vi "sub_generate-ray-casting-grid-map.vi"() -> ()   [LabVIEW 2019]
uses:
  Ctrl/cmd_common.ctl
panel:
  out "oy":dbl[](array[numeric])
  out "ox":dbl[](array[numeric])
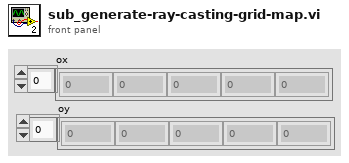
[diagram p1: front panel]
types:
  T1 = typedef "cmd_common.ctl" = enum16{"read", "write"}
  T2 = typedef "NI_Matrix.lvlib/RealMatrix.ctl" = dbl[][]
  T3 = cluster{"resolution":dbl, "EXTEND_AREA":dbl, "MAX_RANGE":dbl, "NP":u32, "NTh":u32, "Q":T2, "R":T2, "Q_sim":T2, "R_sim":T2, "rf_id":cluster{"x":dbl, "y":dbl}[]}
  T4 = cluster{"ox":T2, "oy":T2, "occupancy map":T2, "x_true":T2, "u":T2, "z":T2, "PEst":T2, "min x":dbl, "min y":dbl, "max x":dbl, "max y":dbl, "yw":i32, "xw":i32}
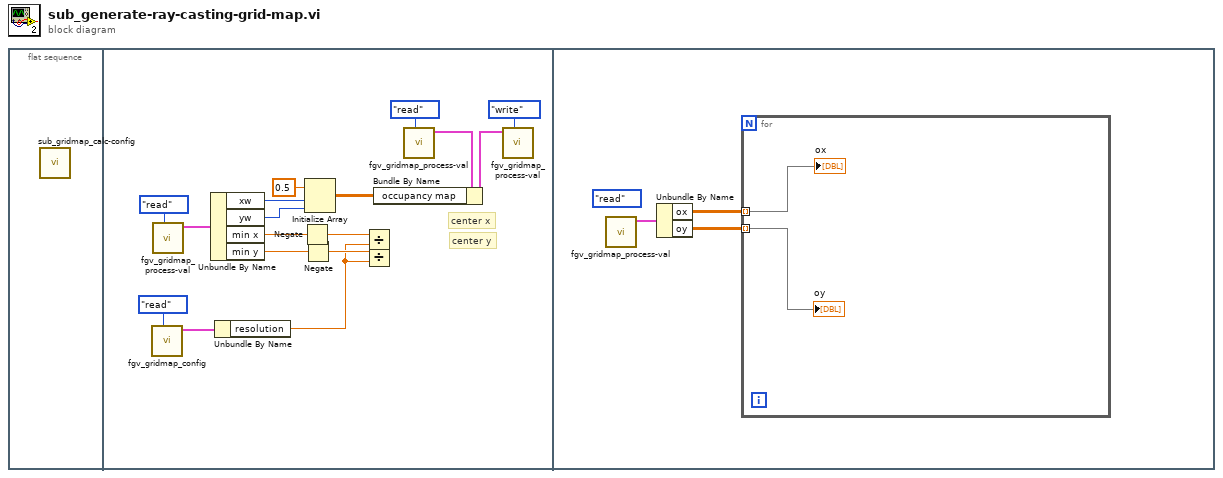
[diagram p0: block diagram]
diagram:
  n1 = flat-sequence {
    frame #0 {
      n2 = call "sub_gridmap_calc-config.vi"() -> ()  [unwired: 12 in]
    }
    frame #1 {
      # "center y"
      # "center x"
      n3 = call "fgv_gridmap_config.vi"("cmd"=cmd_common."read") -> ("pf-val out"=w2:T3)  [unwired: 10 in]
      n4 = call "fgv_gridmap_process-val.vi"("cmd"=cmd_common."read") -> ("p-val  2"=w12:T4)  [unwired: 10 in]
      n5 = Unbundle By Name(w12) -> ("xw"=w11:i32, "yw"=w9:i32, "min x"=w7:dbl, "min y"=w6:dbl)
      n6 = Unbundle By Name(w2) -> ("resolution"=w1:dbl)
      n7 = Negate(x=w7) -> (-x=w5:dbl)
      n8 = Negate(x=w6) -> (-x=w4:dbl)
      n9 = Initialize Array(0.5 ("원소"), w11, w9) -> (w8:dbl[][])
      n10 = Divide(x=w5, y=w1) -> ()  [unwired: 1 out]
      n11 = Divide(x=w4, y=w1) -> ()  [unwired: 1 out]
      n12 = call "fgv_gridmap_process-val.vi"("cmd"=cmd_common."read") -> ("p-val  2"=w17:T4)  [unwired: 10 in]
      n13 = Bundle By Name(cluster=w17, "occupancy map"=w8) -> (w15:T4)
      n14 = call "fgv_gridmap_process-val.vi"("cmd"=cmd_common."write", "p-val"=w15) -> ()  [unwired: 9 in, 1 out]
    }
    frame #2 {
      (unwired) cmd_common."read" ("cmd")
      n15 = call "fgv_gridmap_process-val.vi"() -> ("p-val  2"=w20:T4)  [unwired: 11 in]
      n16 = Unbundle By Name(w20) -> ("ox"=w19:T2, "oy"=w18:T2)
      n17 = for {
        tunnel: w19 -> [w22] mode=indexing
        tunnel: w18 -> [w21] mode=indexing
        "ox" <- w22
        "oy" <- w21
      }
    }
  }
